vi "HRM-close_main.vi"(8 "error in (no error)":errorcluster, 11 "Init cluster":T1) -> (0 "error out":errorcluster)   [LabVIEW 2020]
uses:
  HRM-init_cluster.ctl
  HRM-User_events.ctl
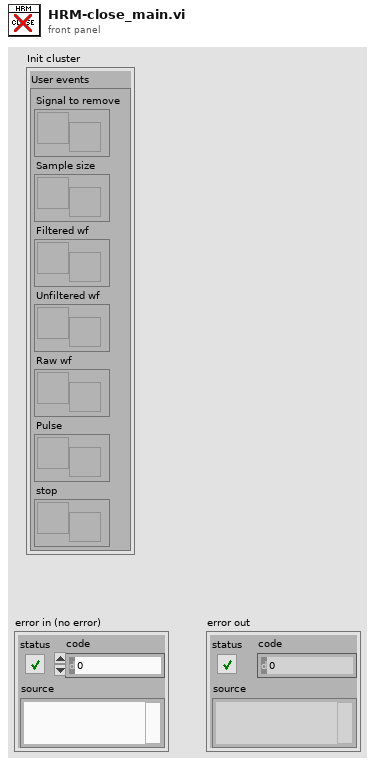
[diagram p1: front panel]
types:
  T1 = typedef "HRM-init_cluster.ctl" = cluster{"User events":T2}
  T2 = typedef "HRM-User_events.ctl" = cluster{"Signal to remove":refnum<user-event>, "Sample size":refnum<user-event>, "Filtered wf":refnum<user-event>, "Unfiltered wf":refnum<user-event>, "Raw wf":refnum<user-event>, "Pulse":refnum<user-event>, "stop":refnum<user-event>}
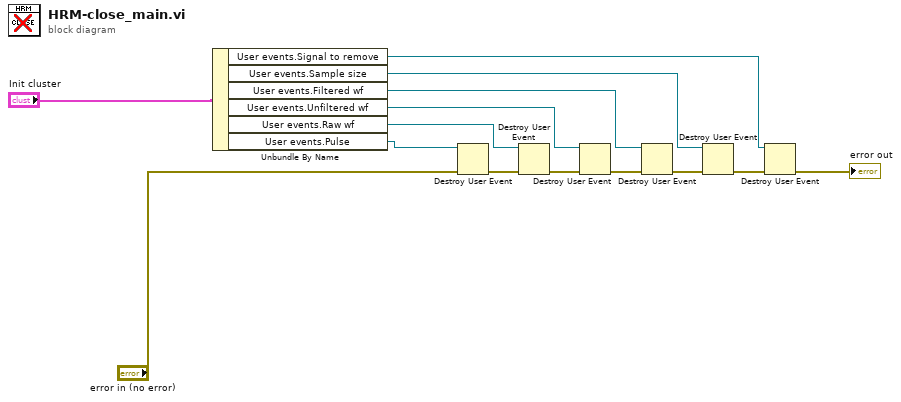
[diagram p0: block diagram]
diagram:
  n1 = Unbundle By Name("Init cluster") -> ("User events.Signal to remove"=w12:refnum<user-event>, "User events.Sample size"=w11:refnum<user-event>, "User events.Filtered wf"=w10:refnum<user-event>, "User events.Unfiltered wf"=w9:refnum<user-event>, "User events.Raw wf"=w8:refnum<user-event>, "User events.Pulse"=w7:refnum<user-event>)
  n2 = Destroy User Event(user event=w7, error in="error in (no error)") -> (error out=w6:errorcluster)
  n3 = Destroy User Event(user event=w8, error in=w6) -> (error out=w2:errorcluster)
  n4 = Destroy User Event(user event=w9, error in=w2) -> (error out=w3:errorcluster)
  n5 = Destroy User Event(user event=w10, error in=w3) -> (error out=w4:errorcluster)
  n6 = Destroy User Event(user event=w11, error in=w4) -> (error out=w5:errorcluster)
  n7 = Destroy User Event(user event=w12, error in=w5) -> (error out=→"error out":errorcluster)
